vi "Close WS.vi"(8 "error in (no error)":errorcluster, 11 "OBS in":refnum<class "OBS.lvclass">) -> (0 "error out":errorcluster, 3 "OBS out":refnum<class "OBS.lvclass">)   [LabVIEW 2020, in "obs-websocket.lvlib" / "OBS.lvclass"]
uses:
  OBS.lvclass
  OBS.lvclass/OBS.ctl
  <vilib>/MediaMongrels Ltd/WebSockets/WebSockets/WebSocket Client/WebSocket Client.lvclass
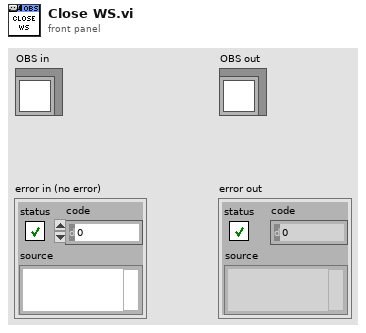
[diagram p1: front panel]
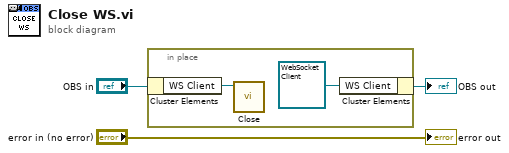
[diagram p0: block diagram]
diagram:
  n1 = in-place {
    n2 = in-place-cluster #1("OBS in") -> ("WS Client"=w5:refnum<class "WebSocket Client.lvclass">)
    n3 = call-dynamic "Close.vi"("WebSocket in"=w5) -> ()  [unwired: 10 in, 1 out]
    n4 = in-place-cluster #1("WS Client"=refnum<class "WebSocket Client.lvclass"> refnum) -> (→"OBS out":refnum<class "OBS.lvclass">)
  }
  "error out" <- "error in (no error)"
